vi "Get GUID.vi"() -> (3 "GUID":string)   [LabVIEW 2014]
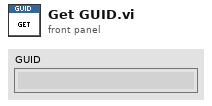
[diagram p1: front panel]
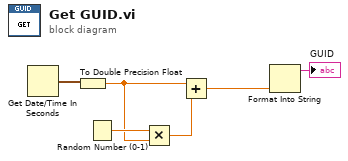
[diagram p0: block diagram]
diagram:
  n1 = Get Date/Time In Seconds() -> (seconds since 1Jan1904=w6:timestamp)
  n2 = To Double Precision Float(number=w6) -> (double precision float=w4:dbl)
  n3 = Random Number (0-1)() -> (number: 0 to 1=w5:dbl)
  n4 = Multiply(x=w5, y=w4) -> (x*y=w3:dbl)
  n5 = Add(x=w4, y=w3) -> (x+y=w2:dbl)
  n6 = Format Into String(w2) -> (resulting string=→"GUID":string)  [unwired: 3 in, 1 out]
